vi "OpenClawTest.vi"(8 "error in":errorcluster, 10 "milliseconds to wait \nfor servo to change":u32=100, 11 "Old Angle":dbl) -> (0 "error out":errorcluster, 1 "FPGA VI Reference Out":T1, 2 "milliseconds to wait \nfor servo to change Out":u32, 3 "New Angle":dbl)   [LabVIEW 2012]
uses:
  FPGA_ref.ctl
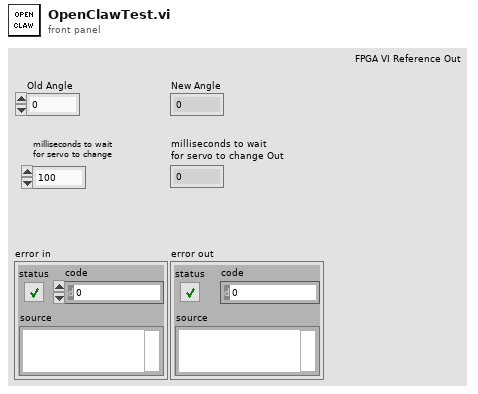
[diagram p1: front panel]
types:
  T1 = typedef "FPGA_ref.ctl" = refnum<k20>
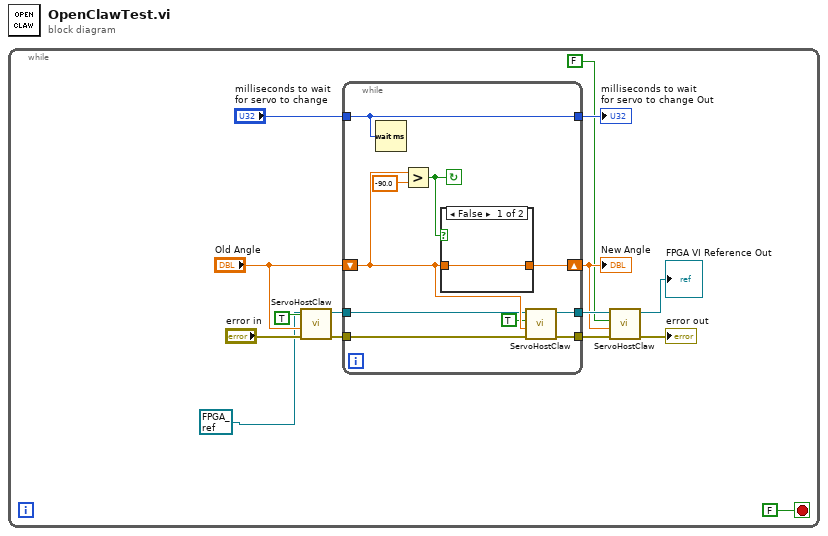
[diagram p0: block diagram]
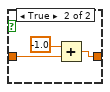
[diagram p2: hidden frame]
diagram:
  n1 = while {
    stop <- FALSE stop-if-true
    n2 = call "ServoHostClaw.vi"("error in"="error in", "Angle (deg) Claw"="Old Angle", 10:TRUE ("Enable"), "FPGA VI Reference In"=T1 refnum) -> ("error out"=w12:errorcluster, "FPGA VI Reference Out"=w13:T1)  [unwired: 6 in]
    n3 = while {
      tunnel: w12 -> [w21]
      shift-right: [w24] -> w4
      shift-left: "Old Angle" -> [w20]
      tunnel: "milliseconds to wait \nfor servo to change" -> [w22]
      tunnel: [w19] -> w6
      tunnel: [w22] -> w14
      tunnel: w13 -> [w18]
      tunnel: [w17] -> w9
      stop <- w23 continue-if-true
      n4 = Wait (ms)(milliseconds to wait=w22) -> ()  [unwired: 1 out]
      n5 = Greater?(x=w20, y=-90.0) -> (0:w23:bool)
      n6 = case shown="False" w23 {
        tunnel: [w26 w28] -> w24
        tunnel: w20 -> [w26 w27]
        frame False {
        }
        frame True {
          n7 = Add(x=-1.0, y=w27) -> (x+y=w28:dbl)
        }
      }
      n8 = call "ServoHostClaw.vi"("error in"=w21, "Angle (deg) Claw"=w20, 10:TRUE ("Enable"), "FPGA VI Reference In"=w18) -> ("error out"=w19:errorcluster, "FPGA VI Reference Out"=w17:T1)  [unwired: 6 in]
    }
    "New Angle" <- w4
    "milliseconds to wait \nfor servo to change Out" <- w14
    n9 = call "ServoHostClaw.vi"("error in"=w6, "Angle (deg) Claw"=w4, 10:FALSE ("Enable"), "FPGA VI Reference In"=w9) -> ("error out"=→"error out":errorcluster, "FPGA VI Reference Out"=→"FPGA VI Reference Out":T1)  [unwired: 6 in]
  }
